vi "Magnet Limits.vi"(0 "instrument.OptiCool":refnum<class "instrument.OptiCool.lvclass">, 5 "Helium (%)":dbl, 7 "Target Field (Oe)":dbl, 9 "Mode":T1, 11 "error in (no error)":errorcluster) -> (4 "instrument.OptiCool out":refnum<class "instrument.OptiCool.lvclass">, 8 "Limited Field (Oe)":dbl, 10 "Mode out":T1, 15 "error out":errorcluster)   [LabVIEW 2019, in "instrument.OptiCool.lvclass"]
uses:
  instrument.OptiCool.lvclass
  <userlib>/LevyLab/Instrument Framework/Instrument Types/Cryostat/Typedefs/Magnet Mode--Enum.ctl
  <userlib>/LevyLab/Instrument Framework/Instrument Types/Cryostat/Instrument.Cryostat.lvclass
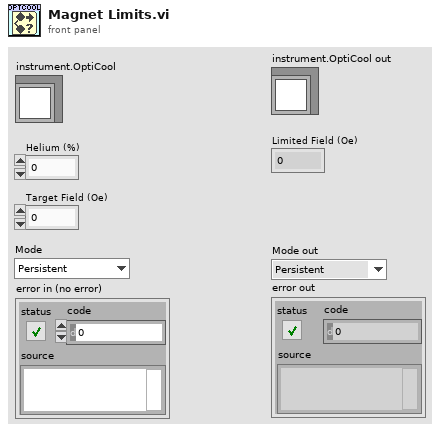
[diagram p1: front panel]
types:
  T1 = typedef "Instrument.Cryostat.lvclass/Magnet Mode--Enum.ctl" = enum16{"Persistent", "Driven"}
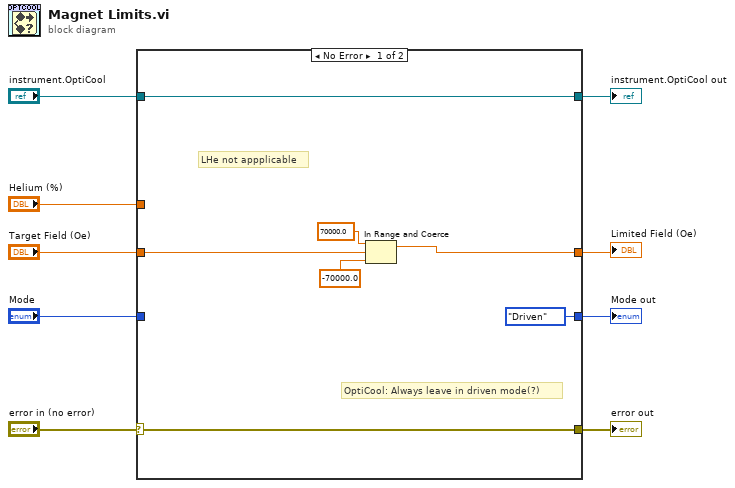
[diagram p0: block diagram]
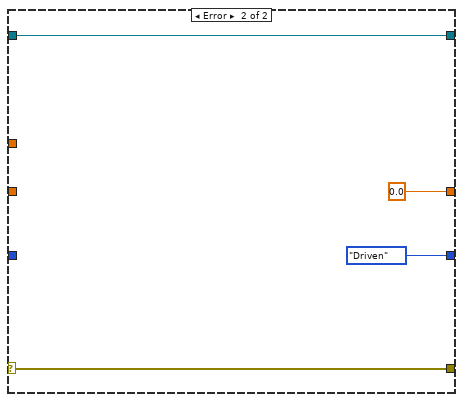
[diagram p2: hidden frame]
diagram:
  n1 = case shown="No Error" "error in (no error)" {
    selector: "error in (no error)" -> [w15 w20]
    tunnel: "Target Field (Oe)" -> [w14 _]
    tunnel: [w13 0.0 ("upper limit")] -> w3
    tunnel: "instrument.OptiCool" -> [w16 w19]
    tunnel: [w16 w19] -> w8
    tunnel: [w15 w20] -> w7
    tunnel: [Magnet_Mode--Enum."Driven" ("Mode") Magnet_Mode--Enum."Driven" ("Mode")] -> w2
    tunnel: "Mode" -> [_ _]
    tunnel: "Helium (%)" -> [_ _]
    frame No Error {
      # "LHe not appplicable"
      # "OptiCool: Always leave in driven mode(?)"
      n2 = In Range and Coerce(upper limit=70000.0, x=w14, lower limit=-70000.0) -> (coerced(x)=w13:dbl)  [unwired: 1 out]
    }
    frame Error {
    }
  }
  "Limited Field (Oe)" <- w3
  "instrument.OptiCool out" <- w8
  "Mode out" <- w2
  "error out" <- w7
